vi "Modbus GUID Lookup.vi"() -> ()   [LabVIEW 2013, in "Modbus Shared.lvlib"]
doc: "Use this Global VI to access the GUIDs assigned to the page resources of the Custom Device."
uses:
  Modbus Shared.lvlib
panel:
  in  "Status Section":string="6dec2bcb-d0f0-4879-8875-bd03842ffe6c"
  in  "Chan Del Prot":string="5f26147a-74dd-4215-ad1d-c30aa09c573d"
  in  "Status":string="d30ff444-76ba-43cf-b605-e86ade14a5f0"
  in  "Custom Device":string="2034df62-bfc7-4efa-9b63-5edc9e07467b"
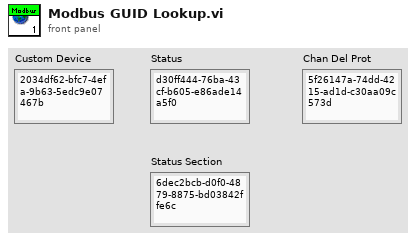
[diagram p1: front panel]
diagram:
